vi "MathFun.vi"(11 "Old Files":T1[](array[typedef])) -> ()   [LabVIEW 2022 SP3]
uses:
  GraphType.ctl
  Curtin1_Label.ctl
panel:
  in  "zoom":bool
  out "names":string[](array[string])
  in  "Set 2":u16(ring) items=["SoundCard2 BabyFace H.AvR", "SoundCard2 BabyFace2 H.AvR", "SoundCard2 BabyFace3 H.AvR", "SoundCard2 DAQ H.AvR", "SoundCard2 DAQ2 H.AvR", "SoundCard2 Focusrite H.AvR", "SoundCard2 Focusrite2 H.AvR", "SoundCard2 Focusrite3 H.AvR", "SoundCard2 ModalShop H.AvR", "SoundCard2 ModalShop2 H.AvR", "SoundCard2 ModalShop3 H.AvR", "SoundCard2 Motu H.AvR", "SoundCard2 Motu2 H.AvR", "SoundCard2 Motu3 H.AvR", "SoundCard2 OctaCapture H.AvR", "SoundCard2 OctaCapture3 H.AvR", "SoundCard2 OctaCapture4 H.AvR"]
  in  "Set 1":u16(ring) items=["SoundCard2 BabyFace H.AvR", "SoundCard2 BabyFace2 H.AvR", "SoundCard2 BabyFace3 H.AvR", "SoundCard2 DAQ H.AvR", "SoundCard2 DAQ2 H.AvR", "SoundCard2 Focusrite H.AvR", "SoundCard2 Focusrite2 H.AvR", "SoundCard2 Focusrite3 H.AvR", "SoundCard2 ModalShop H.AvR", "SoundCard2 ModalShop2 H.AvR", "SoundCard2 ModalShop3 H.AvR", "SoundCard2 Motu H.AvR", "SoundCard2 Motu2 H.AvR", "SoundCard2 Motu3 H.AvR", "SoundCard2 OctaCapture H.AvR", "SoundCard2 OctaCapture3 H.AvR", "SoundCard2 OctaCapture4 H.AvR"]
  in  "Views":T3={"View Type"=0, "Smoothing"=0, "Bands"=0, "Edit"=FALSE, "rescale Y"=FALSE, "rescale X"=FALSE, "X_Low"=0.0, "X_High"=0.0, "dB Range"=40.0, "Excel"=FALSE, "Y Scaling"=FALSE, "X Scaling"=FALSE, "mag/phase 2"=0} {"mag/phase 2" items=["FRF", "rad phase unwrapped", "deg phase unwrapped", "rad phase wrapped", "deg phase wrapped", "White Plots", "MJ Map", "Real and Imaginary"]; "Bands" items=["No Bands", "A Octaves (440-880-1760-3520-7040)", "Curtin Bands (200-780-1740-2930-7000)", "favorites.txt (440)", "JC violin 200-7000 Flat", "JC violin 200-780-1740-2930-7000", "JC violin 200-780-7000", "ObieAlto 200-650-1500-2700-6300 (200-650-1575-2450-6300)"]; "Smoothing" items=["No smoothing"=0, "1/4 semitone"=25, "1/2 semitone"=50, "1 semitone"=100, "2 semitones"=200]; "View Type" items=["As measured"=0, "Normalize"=1, "Cplx Average"=3, "Real Average"=4]}
  out "FRF":cluster{"x0":dbl, "df":dbl, dbl[]}[](graph)
  # "minus"
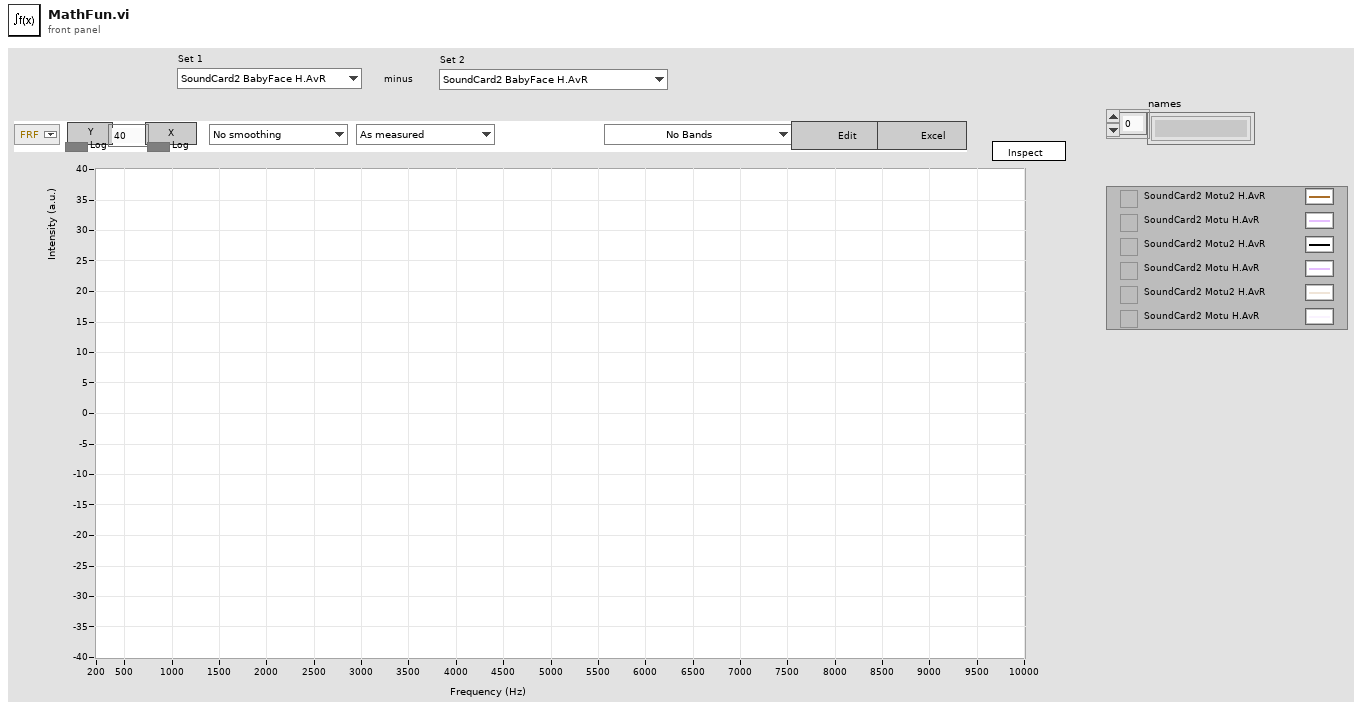
[diagram p1: front panel]
types:
  T1 = typedef "Curtin1_Label.ctl" = cluster{"Show?":bool, "Name":string, "Color":u32, "Path":path, "Show Notes":bool}
  T2 = typedef "GraphType.ctl" = u16
  T3 = cluster{"View Type":u16, "Smoothing":u16, "Bands":u16, "Edit":bool, "rescale Y":bool, "rescale X":bool, "X_Low":dbl, "X_High":dbl, "dB Range":dbl, "Excel":bool, "Y Scaling":bool, "X Scaling":bool, "mag/phase 2":T2}
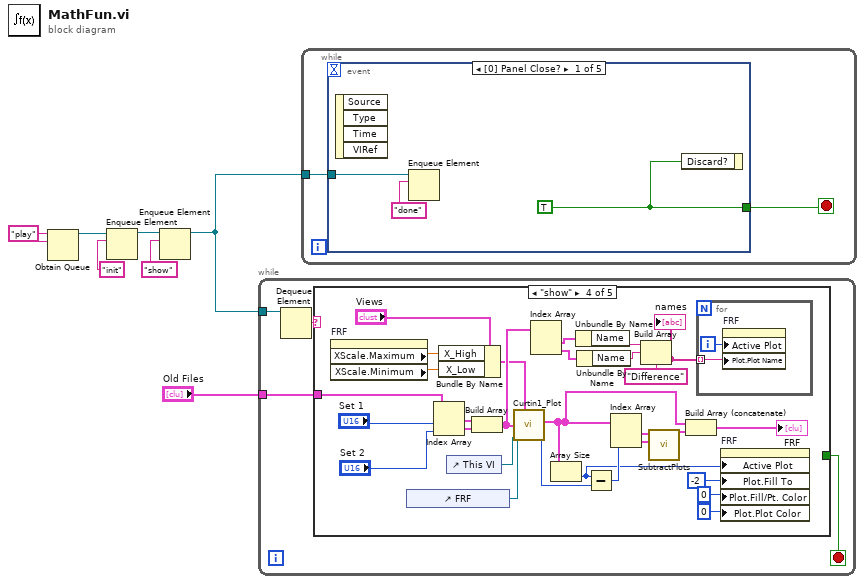
[diagram p0: block diagram]
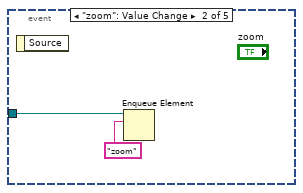
[diagram p2: hidden frame]
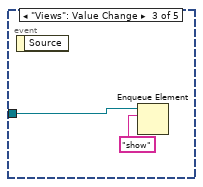
[diagram p3: hidden frame]
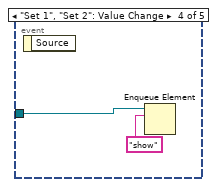
[diagram p4: hidden frame]
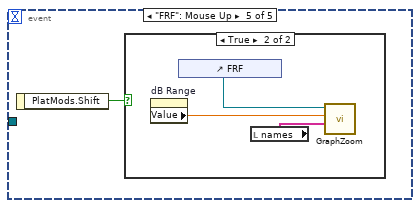
[diagram p5: hidden frame]
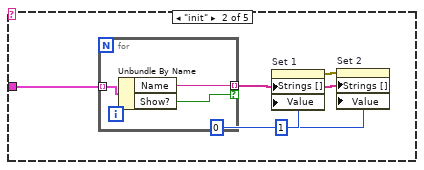
[diagram p8: hidden frame]
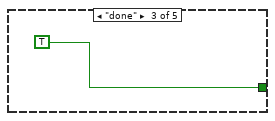
[diagram p9: hidden frame]
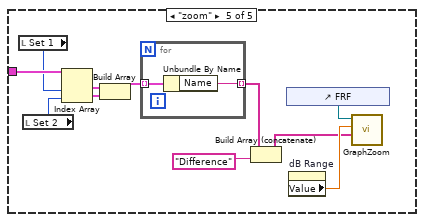
[diagram p10: hidden frame]
diagram:
  w7 = "play" ("name (unnamed)")
  n1 = Obtain Queue(name (unnamed)=w7, element data type=w7) -> (queue out=w2:refnum<queue>)  [unwired: 3 in, 2 out]
  n2 = Enqueue Element(queue=w2, element="init") -> (queue out=w1:refnum<queue>)  [unwired: 2 in, 2 out]
  n3 = Enqueue Element(queue=w1, element="show") -> (queue out=w5:refnum<queue>)  [unwired: 2 in, 2 out]
  n4 = while {
    tunnel: w5 -> [w11]
    tunnel: "Old Files" -> [w8]
    stop <- w9 stop-if-true
    n5 = Dequeue Element(queue=w11) -> (element=w10:string)  [unwired: 2 in, 3 out]
    n6 = case shown="\"show\"" w10 {
      tunnel: [_ _ TRUE _ _] -> w9
      tunnel: w8 -> [_ w16 _ w44 w58]
      frame Default {
      }
      frame "init" {
        n7 = for {
          tunnel: w16 -> [w19] mode=indexing
          tunnel: [w18] -> w14 mode=indexing if=w17
          n8 = Unbundle By Name(w19) -> ("Name"=w18:string, "Show?"=w17:bool)
        }
        n9 = property on="Set 1" class="Ring (strict)"("Strings []"=w14, "Value"=0) -> (error out=w15:errorcluster)  [unwired: 2 in, 1 out]
        n10 = property on="Set 2" class="Ring (strict)"(error in=w15, "Strings []"=w14, "Value"=1) -> ()  [unwired: 1 in, 2 out]
      }
      frame "done" {
      }
      frame "show" {
        n11 = property on="FRF" class="WFGraph (strict)"() -> ("XScale.Maximum"=w22:dbl, "XScale.Minimum"=w21:dbl)  [unwired: 2 in, 2 out]
        n12 = control-ref of="FRF"() -> (w34:refnum<vi>)
        n13 = Index Array(array=w44, index #1="Set 1", index #2="Set 2") -> (element #1=w46:T1, element #2=w45:T1)
        n14 = Bundle By Name(cluster="Views", "X_High"=w22, "X_Low"=w21) -> (w23:T3)
        n15 = control-ref of="This VI"() -> (w49:refnum<vi>)
        n16 = Build Array(w46, w45) -> (w43:T1[])
        n17 = call "Curtin1_Plot.vi"("Settings"=w23, "VI Refnum"=w49, "Files"=w43, "FRF"=w34) -> ("size(s)"=w36:i32, "Average FRF"=w30:cluster{"x0":dbl, "df":dbl, dbl[]}[])  [unwired: 4 in, 2 out]
        n18 = Index Array(array=w43) -> (element #1=w41:T1, element #2=w40:T1)  [unwired: 2 in]
        n19 = Array Size(array=w30) -> (size(s)=w28:i32)
        n20 = Unbundle By Name(w41) -> ("Name"=w39:string)
        n21 = Unbundle By Name(w40) -> ("Name"=w38:string)
        n22 = Subtract(x=w28, y=w36) -> (x-y=w35:i32)
        n23 = Index Array(array=w30, index #1=w35) -> (element #1=w33:cluster{"x0":dbl, "df":dbl, dbl[]}, element #2=w42:cluster{"x0":dbl, "df":dbl, dbl[]})  [unwired: 1 in]
        n24 = Build Array(w39, w38, "Difference" ("element")) -> (w37:string[])
        "names" <- w37
        n25 = call "SubtractPlots.vi"("Set 2"=w42, "Set 1"=w33) -> ("Difference"=w32:cluster{"x0":dbl, "df":dbl, dbl[]})  [unwired: 9 in]
        n26 = Build Array (concatenate)(w30, w32) -> (→"FRF":cluster{"x0":dbl, "df":dbl, dbl[]}[])
        n27 = for {
          tunnel: w37 -> [w51] mode=indexing
          i -> [w50]
          n28 = property on="FRF" class="WFGraph (strict)"("Active Plot"=w50, "Plot.Plot Name"=w51) -> ()  [unwired: 2 in, 2 out]
        }
        n29 = property on="FRF" class="WFGraph (strict)"("Active Plot"=w28, "Plot.Fill To"=i16 -2, "Plot.Fill/Pt. Color"=u32 0 ("Plot.Fill/Point Color"), "Plot.Plot Color"=u8 0 ("Plot.Line Style")) -> ()  [unwired: 2 in, 2 out]
      }
      frame "zoom" {
        n30 = local read "Set 1"() -> (w56:u16)
        n31 = local read "Set 2"() -> (w55:u16)
        n32 = Index Array(array=w58, index #1=w56, index #2=w55) -> (element #1=w60:T1, element #2=w59:T1)
        n33 = Build Array(w60, w59) -> (w57:T1[])
        n34 = for {
          tunnel: w57 -> [w64] mode=indexing
          tunnel: [w63] -> w54 mode=indexing
          n35 = Unbundle By Name(w64) -> ("Name"=w63:string)
        }
        n36 = Build Array (concatenate)(w54, "Difference") -> (w53:string[])
        n37 = control-ref of="FRF"() -> (w61:refnum<vi>)
        n38 = property on="dB Range" class="DigNum (strict)"() -> ("Value"=w62:dbl)  [unwired: 2 in, 2 out]
        n39 = call "GraphZoom.vi"("Names"=w53, "dB Range"=w62, "Graph"=w61) -> ()  [unwired: 9 in]
      }
    }
  }
  n40 = while {
    tunnel: w5 -> [w65]
    stop <- w66 stop-if-true
    n41 = event shown="[0] Panel Close?" {
      selector: _ -> [_ _ _ _ _]
      dyn-events: _ -> [_ _ _ _ _]
      timeout: _ -> [_ _ _ _ _]
      tunnel: [w67 _ _ _ _] -> w66
      tunnel: w65 -> [w68 w70 w72 w74 _]
      event Panel Close? {
        w67 = TRUE
        n42 = event-data() -> ()  [unwired: 1 in, 4 out]
        n43 = Enqueue Element(queue=w68, element="done") -> ()  [unwired: 2 in, 3 out]
        n44 = event-data("Discard?"=w67) -> ()  [unwired: 1 in, 1 out]
      }
      event "zoom": Value Change {
        n45 = event-data() -> ()  [unwired: 1 in, 1 out]
        n46 = Enqueue Element(queue=w70, element="zoom") -> ()  [unwired: 2 in, 3 out]
      }
      event "Views": Value Change {
        n47 = event-data() -> ()  [unwired: 1 in, 1 out]
        n48 = Enqueue Element(queue=w72, element="show") -> ()  [unwired: 2 in, 3 out]
      }
      event "Set 1", "Set 2": Value Change {
        n49 = event-data() -> ()  [unwired: 1 in, 1 out]
        n50 = Enqueue Element(queue=w74, element="show") -> ()  [unwired: 2 in, 3 out]
      }
      event "FRF": Mouse Up {
        n51 = event-data() -> ("PlatMods.Shift"=w76:bool)  [unwired: 1 in]
        n52 = case shown="True" w76 {
          frame False {
          }
          frame True {
            n53 = property on="dB Range" class="DigNum (strict)"() -> ("Value"=w78:dbl)  [unwired: 2 in, 2 out]
            n54 = control-ref of="FRF"() -> (w79:refnum<vi>)
            n55 = local read "names"() -> (w77:string[])
            n56 = call "GraphZoom.vi"("Names"=w77, "dB Range"=w78, "Graph"=w79) -> ()  [unwired: 9 in]
          }
        }
      }
    }
  }
